vi "Continuous Serial Write and Read.vi"() -> ()   [LabVIEW 2017]
doc: "This example performs writes and reads on a serial port, as directed by the user. You can press the Write and Read buttons, and change the Read Count, while the example is running.\n\nThe parameters set for the serial port must match the parameters of the connected instrument or device. In this example, the Read Count parameter specifies the number of bytes that the serial port reads. If there were more bytes at the port than the specified number, those bytes would not be read. If there were less bytes at the port than the specified number, you would receive a timeout error.\n\nThis example expands upon the flow control options for XON and XOFF, allowing the user to choose those control characters. Also, the user can enable or disable a termination character. Some devices require a termination character in order to identify the end of command strings. Some devices send a termination character to signify the end of data to be read. This example shows how you can end the Read operation once a termination character is detected in the buffer and/or append a termination character at the end of the Write data."
uses:
  Program Files (x86)/National Instruments/LabVIEW 2017/examples/Instrument IO/Serial/support/Serial - Settings.ctl
  Program Files (x86)/National Instruments/LabVIEW 2017/examples/Instrument IO/Serial/support/Serial - XON-XOFF Characters.ctl
  Program Files (x86)/National Instruments/LabVIEW 2017/examples/Instrument IO/Serial/support/Serial - ASCII Characters.ctl
  <vilib>/Instr/_visa.llb/VISA Configure Serial Port (Instr).vi
panel:
  out "Intensity Graph 2":i32[][](graph)
  out "Color Box 17":u32(colorbox)
  out "Color Box 16":u32(colorbox)
  out "Color Box 15":u32(colorbox)
  out "Color Box 14":u32(colorbox)
  out "Color Box 13":u32(colorbox)
  out "Color Box 12":u32(colorbox)
  out "Color Box 11":u32(colorbox)
  out "Color Box 10":u32(colorbox)
  out "Color Box 9":u32(colorbox)
  out "Color Box 8":u32(colorbox)
  out "Color Box 7":u32(colorbox)
  out "Color Box 6":u32(colorbox)
  out "Color Box 5":u32(colorbox)
  out "Color Box 4":u32(colorbox)
  out "Color Box 3":u32(colorbox)
  out "Color Box 2":u32(colorbox)
  out "Numeric":dbl
  in  "End Write on Termination Character?":bool=TRUE
  in  "Stop":bool
  in  "Read Count":u32=1000
  out "Response":string
  in  "XON/XOFF Characters":T1={"XON"=enum."DC1", "XOFF"=enum."DC3"}
  in  "Serial Settings":T3={"baud rate"=9600, "data bits"=8, "parity"=enum."None", "stop bits"=10, "flow control"=0} {"flow control" items=["None"=0, "XON/XOFF"=1, "RTS/CTS"=2, "DTR/DSR"=4]; "stop bits" items=["1.0"=10, "1.5"=15, "2.0"=20]; "data bits" min=5 max=8 step=1; "baud rate" items=["75"=75, "110"=110, "134"=134, "150"=150, "300"=300, "600"=600, "1200"=1200, "1800"=1800, "2400"=2400, "4800"=4800, "7200"=7200, "9600"=9600, "14400"=14400, "19200"=19200, "28800"=28800, "38400"=38400, "56000"=56000, "57600"=57600, "115200"=115200, "128000"=128000, "230400"=230400]}
  in  "End Read on Termination Character?":bool=TRUE
  in  "VISA resource name":refnum<visa-resource-name>="COM1"
  # "Overview: Demonstrates the use of the VISA functions to write commands to and read responses from a serial instrument continuously in a loop.\nRequirements: NI-VISA Driver\nInstructions:\n1. Run the VI.\n2. Specify a Command and click the Write button.\n3. Read a Response by clicking the Read button.\n4. Click Stop to stop the VI."
  # "0xA is equivalent to a '\\n' character, which is a line feed."
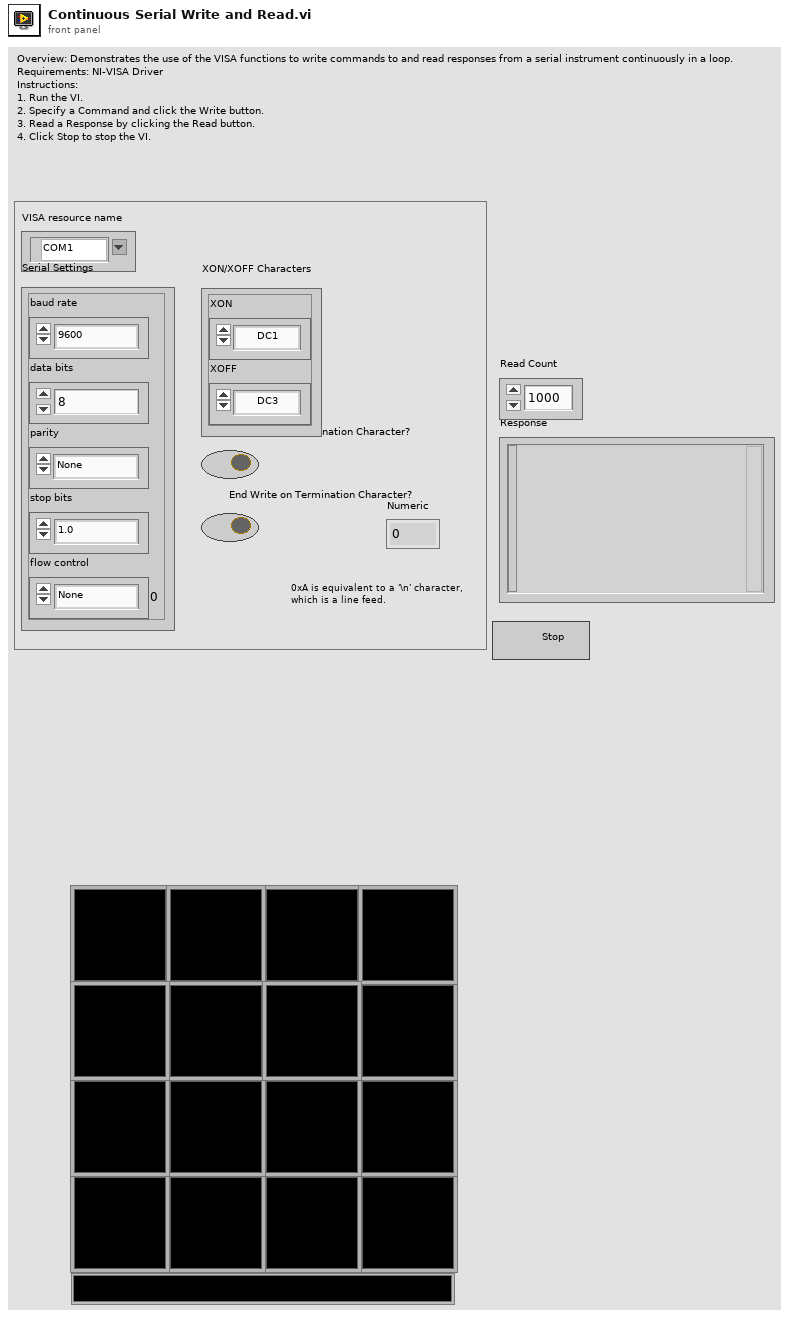
[diagram p1: front panel]
types:
  T1 = typedef "Serial - XON-XOFF Characters.ctl" = cluster{"XON":T2, "XOFF":T2}
  T2 = typedef "Serial - ASCII Characters.ctl" = enum16{"NUL", "SOH", "STX", "ETX", "EOT", "ENQ", "ACK", "BEL", "BS", "HT", "LF", "VT", "FF", "CR", "SO", "SI", "DLE", "DC1", "DC2", "DC3", "DC4", "NAK", "SYN", "ETB", "CAN", "EM", "SUB", "ESC", "FS", "GS", "RS", "US", "SP", "!", "\"", "#", "$", "%", "&", "'", "(", ")", "*", "+", ",", "- (-)", ".", "/", "0", "1", "2", "3", "4", "5", "6", "7", "8", "9", ":", ";", "<", "=", ">", "?", "@", "A", "B", "C", "D", "E", "F", "G", "H", "I", "J", "K", "L", "M", "N", "O", "P", "Q", "R", "S", "T", "U", "V", "W", "X", "Y", "Z", "[", "\\", "]", "^", "_", "`", "a", "b", "c", "d", "e", "f", "g", "h", "i", "j", "k", "l", "m", "n", "o", "p", "q", "r", "s", "t", "u", "v", "w", "x", "y", "z", "{", "|", "}", "~"}
  T3 = typedef "Serial - Settings.ctl" = cluster{"baud rate":u32, "data bits":u16, "parity":enum16{"None", "Odd", "Even", "Mark", "Space"}, "stop bits":u16, "flow control":u16}
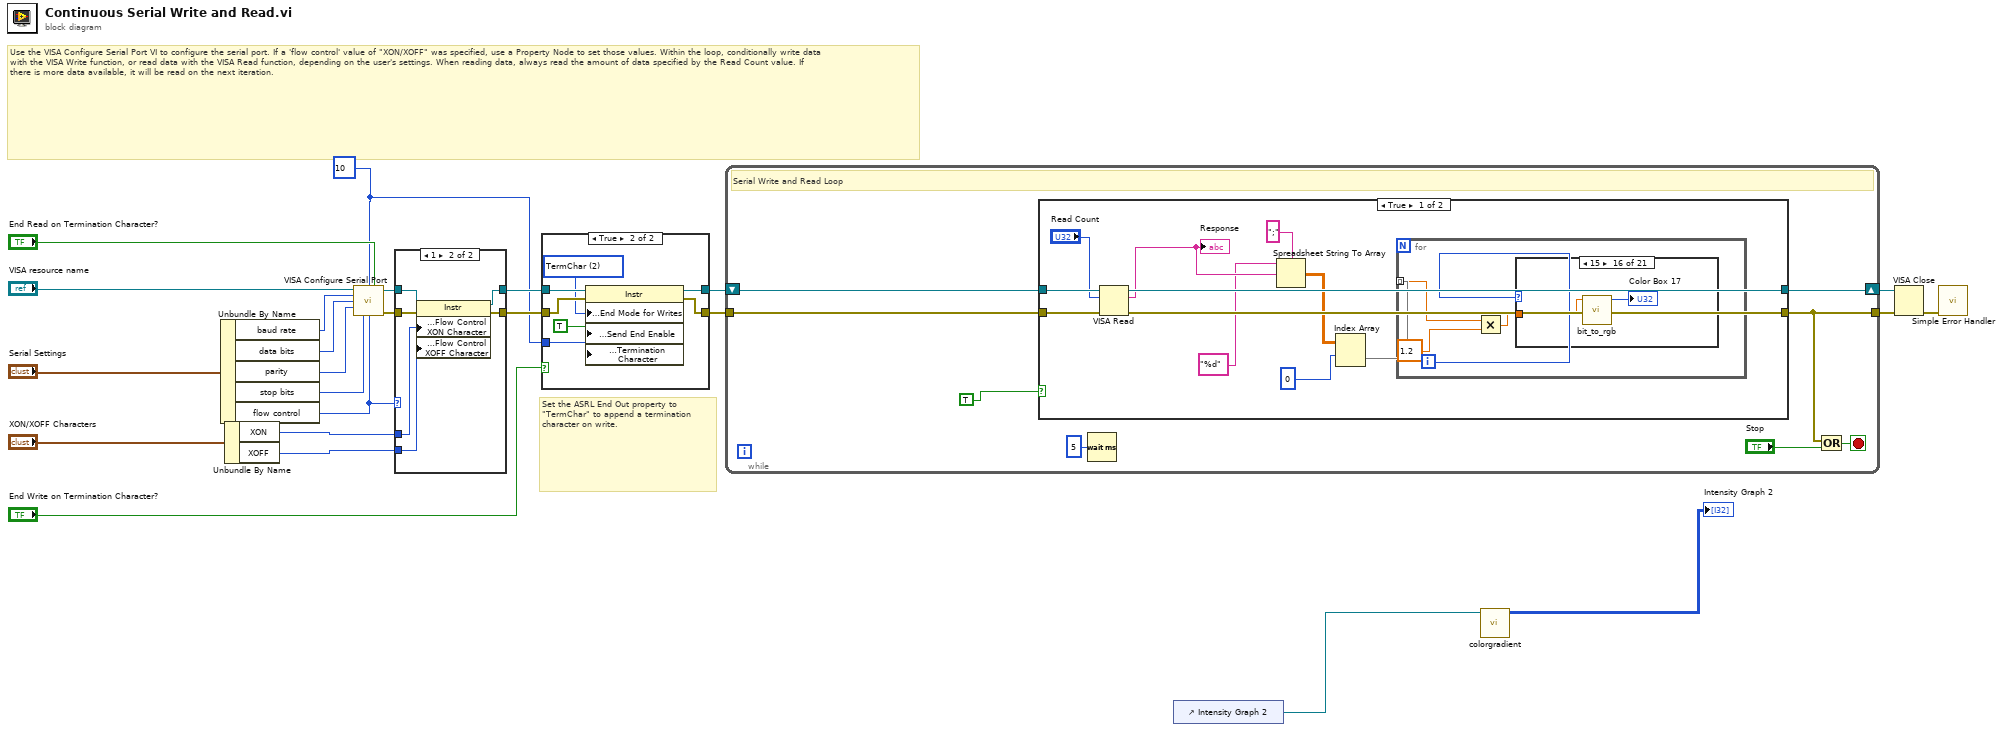
[diagram p0: block diagram]
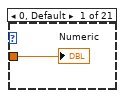
[diagram p4: hidden frame]
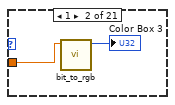
[diagram p5: hidden frame]
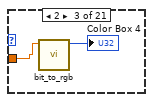
[diagram p6: hidden frame]
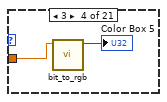
[diagram p7: hidden frame]
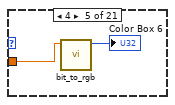
[diagram p8: hidden frame]
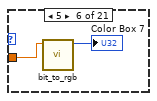
[diagram p9: hidden frame]
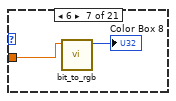
[diagram p10: hidden frame]
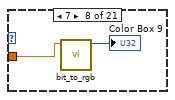
[diagram p11: hidden frame]
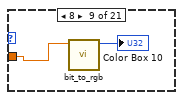
[diagram p12: hidden frame]
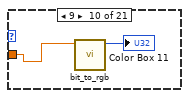
[diagram p13: hidden frame]
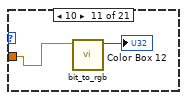
[diagram p14: hidden frame]
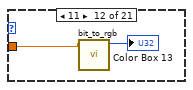
[diagram p15: hidden frame]
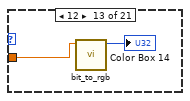
[diagram p16: hidden frame]
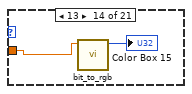
[diagram p17: hidden frame]
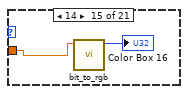
[diagram p18: hidden frame]
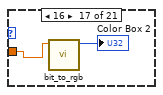
[diagram p19: hidden frame]
diagram:
  w3 = 10
  # "Set the ASRL End Out property to \"TermChar\" to append a termination character on write."
  # "Use the VISA Configure Serial Port VI to configure the serial port. If a 'flow control' value of \"XON/XOFF\" was specified, use a Property Node to set those values. Within the loop, conditionally write data with the VISA Write function, or read data with the VISA Read function, depending on the user's settings. When reading data, always read the amount of data specified by the Read Count value. If there is more data available, it will be read on the next iteration."
  n1 = Unbundle By Name("Serial Settings") -> ("baud rate"=w17:u32, "data bits"=w18:u16, "parity"=w19:enum16{"None", "Odd", "Even", "Mark", "Space"}, "stop bits"=w20:u16, "flow control"=w11:u16)
  n2 = Unbundle By Name("XON/XOFF Characters") -> ("XON"=w10:T2, "XOFF"=w9:T2)
  n3 = call-poly "VISA Configure Serial Port"("VISA resource name"="VISA resource name", "termination char\n(0xA = '\\n' = LF)"=w3, "Enable Termination\nChar (T)"="End Read on Termination Character?", "baud rate (9600)"=w17, "data bits (8)"=w18, "parity (0:none)"=w19, "stop bits (10: 1 bit)"=w20, "flow control (0:none)"=w11) -> ("VISA resource name out"=w21:refnum<visa-resource-name>, "error out"=w22:errorcluster)  [unwired: 2 in, 4 out]
  n4 = case shown="1" w11 {
    tunnel: [w25 w32] -> w8
    tunnel: [w26 w31] -> w6
    tunnel: w22 -> [w25 w30]
    tunnel: w21 -> [w26 w29]
    tunnel: w10 -> [_ w28]
    tunnel: w9 -> [_ w27]
    frame Default {
    }
    frame 1 {
      n5 = property class="Instr"(reference=w29, error in=w30, "Serial Settings:Flow Control XON Character"=w28, "Serial Settings:Flow Control XOFF Character"=w27) -> (reference out=w31:refnum<visa-resource-name>, error out=w32:errorcluster)
    }
  }
  n6 = case shown="True" "End Write on Termination Character?" {
    tunnel: w6 -> [w33 w41]
    tunnel: w8 -> [w34 w40]
    tunnel: [w33 w39] -> w5
    tunnel: [w34 w38] -> w7
    tunnel: w3 -> [_ w36]
    frame False {
    }
    frame True {
      w37 = u16 2 items=["None", "LastBit", "TermChar", "Break"] ("Serial Settings:Serial End Mode for Writes")
      n7 = property class="Instr"(reference=w41, error in=w40, "Serial Settings:End Mode for Writes"=w37, "Message Based Settings:Send End Enable"=TRUE, "Message Based Settings:Termination Character"=w36) -> (reference out=w39:refnum<visa-resource-name>, error out=w38:errorcluster)
    }
  }
  n8 = while {
    shift-right: [w49] -> w12
    shift-left: w5 -> [w48]
    tunnel: w7 -> [w47]
    tunnel: [w44] -> w13
    stop <- w45 stop-if-true
    # "Serial Write and Read Loop"
    n9 = case shown="True" TRUE {
      tunnel: [w58 w99] -> w49
      tunnel: w48 -> [w60 w99]
      tunnel: [w56 w98] -> w44
      tunnel: w47 -> [w59 w98]
      frame True {
        n10 = VISA Read(VISA resource name=w60, byte count="Read Count", error in (no error)=w59) -> (VISA resource name out=w58:refnum<visa-resource-name>, read buffer=w55:string, error out=w56:errorcluster)  [unwired: 1 out]
        "Response" <- w55
        n11 = Spreadsheet String To Array(delimiter (Tab)=";", format string="%d", spreadsheet string=w55) -> (array=w52:dbl[][])  [unwired: 1 in]
        n12 = Index Array(array=w52, index (row)=0) -> (element=w50:dbl[])  [unwired: 1 in]
        n13 = for {
          tunnel: w50 -> [w62] mode=indexing
          i -> [w64]
          n14 = Multiply(x=w62, y=1.2) -> (x*y=w61:dbl)
          n15 = case shown="15" w64 {
            tunnel: w61 -> [w65 w66 w68 w70 w72 w74 w76 w78 w80 w82 w84 w86 w88 w90 w92 w94 w96 _ _ _ _]
            frame 0, Default {
              "Numeric" <- w65
            }
            frame 1 {
              n16 = call "bit_to_rgb.vi"("Slide"=w66) -> ("Color"=→"Color Box 3":u32)  [unwired: 10 in]
            }
            frame 2 {
              n17 = call "bit_to_rgb.vi"("Slide"=w68) -> ("Color"=→"Color Box 4":u32)  [unwired: 10 in]
            }
            frame 3 {
              n18 = call "bit_to_rgb.vi"("Slide"=w70) -> ("Color"=→"Color Box 5":u32)  [unwired: 10 in]
            }
            frame 4 {
              n19 = call "bit_to_rgb.vi"("Slide"=w72) -> ("Color"=→"Color Box 6":u32)  [unwired: 10 in]
            }
            frame 5 {
              n20 = call "bit_to_rgb.vi"("Slide"=w74) -> ("Color"=→"Color Box 7":u32)  [unwired: 10 in]
            }
            frame 6 {
              n21 = call "bit_to_rgb.vi"("Slide"=w76) -> ("Color"=→"Color Box 8":u32)  [unwired: 10 in]
            }
            frame 7 {
              n22 = call "bit_to_rgb.vi"("Slide"=w78) -> ("Color"=→"Color Box 9":u32)  [unwired: 10 in]
            }
            frame 8 {
              n23 = call "bit_to_rgb.vi"("Slide"=w80) -> ("Color"=→"Color Box 10":u32)  [unwired: 10 in]
            }
            frame 9 {
              n24 = call "bit_to_rgb.vi"("Slide"=w82) -> ("Color"=→"Color Box 11":u32)  [unwired: 10 in]
            }
            frame 10 {
              n25 = call "bit_to_rgb.vi"("Slide"=w84) -> ("Color"=→"Color Box 12":u32)  [unwired: 10 in]
            }
            frame 11 {
              n26 = call "bit_to_rgb.vi"("Slide"=w86) -> ("Color"=→"Color Box 13":u32)  [unwired: 10 in]
            }
            frame 12 {
              n27 = call "bit_to_rgb.vi"("Slide"=w88) -> ("Color"=→"Color Box 14":u32)  [unwired: 10 in]
            }
            frame 13 {
              n28 = call "bit_to_rgb.vi"("Slide"=w90) -> ("Color"=→"Color Box 15":u32)  [unwired: 10 in]
            }
            frame 14 {
              n29 = call "bit_to_rgb.vi"("Slide"=w92) -> ("Color"=→"Color Box 16":u32)  [unwired: 10 in]
            }
            frame 15 {
              n30 = call "bit_to_rgb.vi"("Slide"=w94) -> ("Color"=→"Color Box 17":u32)  [unwired: 10 in]
            }
            frame 16 {
              n31 = call "bit_to_rgb.vi"("Slide"=w96) -> ("Color"=→"Color Box 2":u32)  [unwired: 10 in]
            }
            frame 17 {
            }
            frame 18 {
            }
            frame 19 {
            }
            frame 20 {
            }
          }
        }
      }
      frame False {
      }
    }
    n32 = Wait (ms)(milliseconds to wait=u32 5) -> ()  [unwired: 1 out]
    n33 = Or(x=w44, y="Stop") -> (x .or. y?=w45:bool)
  }
  n34 = control-ref of="Intensity Graph 2"() -> (w1:refnum<vi>)
  n35 = call "colorgradient.vi"("IntensityGraph in"=w1) -> ("Array"=→"Intensity Graph 2":i32[][])  [unwired: 10 in]
  n36 = VISA Close(VISA resource name=w12, error in (no error)=w13) -> (error out=w14:errorcluster)
  n37 = call <vilib>:"Simple Error Handler.vi"("error in (no error)"=w14) -> ()  [unwired: 1 in, 8 out]
